vi "PEXPIREAT.vi"(8 "error in (no error)":errorcluster, 9 "expire time":timestamp, 10 "key":string, 11 "Redis Client in":refnum<class "Redis Client.lvclass">) -> (0 "error out":errorcluster, 2 "expire set?":bool, 3 "Redis Client out":refnum<class "Redis Client.lvclass">)   [LabVIEW 2019, in "Redis Client for LabVIEW.lvlib" / "Redis Client.lvclass"]
uses:
  Redis Client.lvclass
  lib/RESP3-for-LabVIEW/RESP3/subVIs/RESP3 Make String Base.vi
  lib/RESP3-for-LabVIEW/RESP3/types/RESP3 data type attribute.vi
  lib/RESP3-for-LabVIEW/RESP3/high-level/RESP3 Make Array.vi
  lib/RESP3-for-LabVIEW/RESP3/high-level/RESP3 Get String.vi
  lib/RESP3-for-LabVIEW/RESP3/high-level/RESP3 Get Integer.vi
  lib/RESP3-for-LabVIEW/RESP3/RESP3.lvlib
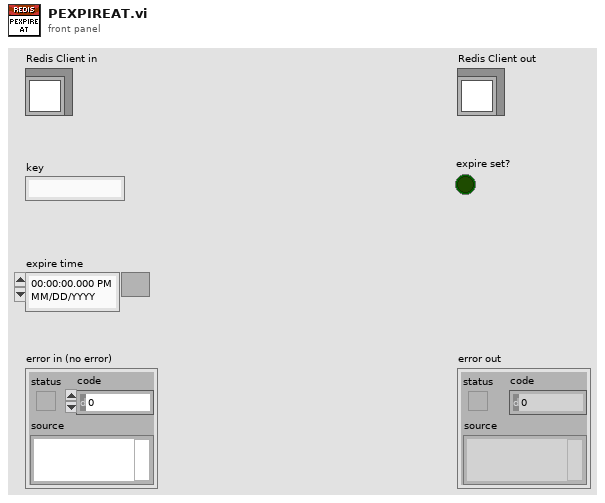
[diagram p1: front panel]
types:
  T1 = typedef "RESP3.lvlib/RESP3 Type.ctl" = enum8{"<0x00>", "<0x01>", "<0x02>", "<0x03>", "<0x04>", "<0x05>", "<0x06>", "<0x07>", "<0x08>", "<0x09>", "<0x0A>", "<0x0B>", "<0x0C>", "<0x0D>", "<0x0E>", "<0x0F>", "<0x10>", "<0x11>", "<0x12>", "<0x13>", "<0x14>", "<0x15>", "<0x16>", "<0x17>", "<0x18>", "<0x19>", "<0x1A>", "<0x1B>", "<0x1C>", "<0x1D>", "<0x1E>", "<0x1F>", "\" \"", "BLOB ERROR", "\"\"\"", "BOOLEAN", "BLOB", "MAP", "\"&\"", "\"'\"", "BIG NUMBER", "\")\"", "ARRAY", "STRING", "DOUBLE", "ERROR", "END", "\"/\"", "\"0\"", "\"1\"", "\"2\"", "\"3\"", "\"4\"", "\"5\"", "\"6\"", "\"7\"", "\"8\"", "\"9\"", "INTEGER", "STREAM", "\"<\"", "VERBATIM STRING", "PUSH", "\"?\"", "\"@\"", "\"A\"", "\"B\"", "\"C\"", "\"D\"", "\"E\"", "\"F\"", "\"G\"", "\"H\"", "\"I\"", "\"J\"", "\"K\"", "\"L\"", "\"M\"", "\"N\"", "\"O\"", "\"P\"", "\"Q\"", "\"R\"", "\"S\"", "\"T\"", "\"U\"", "\"V\"", "\"W\"", "\"X\"", "\"Y\"", "\"Z\"", "\"[\"", "\"\\\"", "\"]\"", "\"^\"", "NULL", "\"`\"", "\"a\"", "\"b\"", "\"c\"", "\"d\"", "\"e\"", "\"f\"", "\"g\"", "\"h\"", "\"i\"", "\"j\"", "\"k\"", "\"l\"", "\"m\"", "\"n\"", "\"o\"", "\"p\"", "\"q\"", "\"r\"", "\"s\"", "\"t\"", "\"u\"", "\"v\"", "\"w\"", "\"x\"", "\"y\"", "\"z\"", "\"{\"", "ATTRIBUTES", "\"}\"", "SET", "<0x7F>", "<0x80>", "<0x81>", "<0x82>", "<0x83>", "<0x84>", "<0x85>", "<0x86>", "<0x87>", "<0x88>", "<0x89>", "<0x8A>", "<0x8B>", "<0x8C>", "<0x8D>", "<0x8E>", "<0x8F>", "<0x90>", "<0x91>", "<0x92>", "<0x93>", "<0x94>", "<0x95>", "<0x96>", "<0x97>", "<0x98>", "<0x99>", "<0x9A>", "<0x9B>", "<0x9C>", "<0x9D>", "<0x9E>", "<0x9F>", "<0xA0>", "<0xA1>", "<0xA2>", "<0xA3>", "<0xA4>", "<0xA5>", "<0xA6>", "<0xA7>", "<0xA8>", "<0xA9>", "<0xAA>", "<0xAB>", "<0xAC>", "<0xAD>", "<0xAE>", "<0xAF>", "<0xB0>", "<0xB1>", "<0xB2>", "<0xB3>", "<0xB4>", "<0xB5>", "<0xB6>", "<0xB7>", "<0xB8>", "<0xB9>", "<0xBA>", "<0xBB>", "<0xBC>", "<0xBD>", "<0xBE>", "<0xBF>", "<0xC0>", "<0xC1>", "<0xC2>", "<0xC3>", "<0xC4>", "<0xC5>", "<0xC6>", "<0xC7>", "<0xC8>", "<0xC9>", "<0xCA>", "<0xCB>", "<0xCC>", "<0xCD>", "<0xCE>", "<0xCF>", "<0xD0>", "<0xD1>", "<0xD2>", "<0xD3>", "<0xD4>", "<0xD5>", "<0xD6>", "<0xD7>", "<0xD8>", "<0xD9>", "<0xDA>", "<0xDB>", "<0xDC>", "<0xDD>", "<0xDE>", "<0xDF>", "<0xE0>", "<0xE1>", "<0xE2>", "<0xE3>", "<0xE4>", "<0xE5>", "<0xE6>", "<0xE7>", "<0xE8>", "<0xE9>", "<0xEA>", "<0xEB>", "<0xEC>", "<0xED>", "<0xEE>", "<0xEF>", "<0xF0>", "<0xF1>", "<0xF2>", "<0xF3>", "<0xF4>", "<0xF5>", "<0xF6>", "<0xF7>", "<0xF8>", "<0xF9>", "<0xFA>", "<0xFB>", "<0xFC>", "<0xFD>", "<0xFE>"}
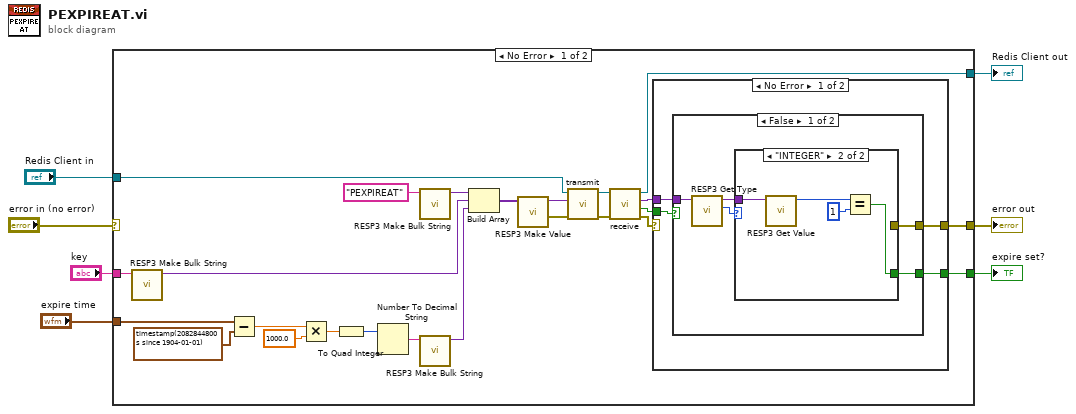
[diagram p0: block diagram]
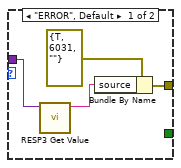
[diagram p2: hidden frame]
diagram:
  n1 = case shown="No Error" "error in (no error)" {
    selector: "error in (no error)" -> [_ w51]
    tunnel: [w29 w51] -> w6
    tunnel: "Redis Client in" -> [w31 w50]
    tunnel: [w30 w50] -> w4
    tunnel: "key" -> [w18 _]
    tunnel: [w19 _] -> w1
    tunnel: "expire time" -> [w12 _]
    frame No Error {
      n2 = call "RESP3 Make Bulk String.vi"("String"=w18) -> ("RESP3 Value out"=w17:variant)  [unwired: 9 in, 1 out]
      n3 = Subtract(x=w12, y=timestamp(2082844800 s since 1904-01-01)) -> (x-y=w11:dbl)
      n4 = Multiply(x=w11, y=1000.0) -> (x*y=w10:dbl)
      n5 = To Quad Integer(1:w10) -> (0:w8:i64)
      n6 = Number To Decimal String(number=w8) -> (decimal integer string=w15:string)  [unwired: 1 in]
      n7 = call "RESP3 Make Bulk String.vi"("String"="PEXPIREAT" ("string in")) -> ("RESP3 Value out"=w20:variant)  [unwired: 9 in, 1 out]
      n8 = call "RESP3 Make Bulk String.vi"("String"=w15) -> ("RESP3 Value out"=w16:variant)  [unwired: 9 in, 1 out]
      n9 = Build Array(w20, w17, w16) -> (w14:variant[])
      n10 = call-poly "RESP3 Make Value.vi"("RESP3 Values in"=w14) -> ("error out"=w23:errorcluster, "RESP3 Value out"=w22:variant)  [unwired: 9 in]
      n11 = call-dynamic "transmit.vi"("error in (no error)"=w23, "RESP3 Value"=w22, "Redis Client in"=w31) -> ("error out"=w27:errorcluster, "Redis Client out"=w28:refnum<class "Redis Client.lvclass">)  [unwired: 7 in]
      n12 = call-dynamic "receive.vi"("error in (no error)"=w27, "Redis Client in"=w28) -> ("error out"=w24:errorcluster, "timed out?"=w25:bool, "RESP3 Value"=w26:variant, "Redis Client out"=w30:refnum<class "Redis Client.lvclass">)  [unwired: 6 in]
      n13 = case shown="No Error" w24 {
        selector: w24 -> [_ w49]
        tunnel: [w35 w49] -> w29
        tunnel: w26 -> [w34 _]
        tunnel: w25 -> [w33 _]
        tunnel: [w32 _] -> w19
        frame No Error {
          n14 = case shown="False" w33 {
            tunnel: [w40 _] -> w35
            tunnel: w34 -> [w38 _]
            tunnel: [w36 _] -> w32
            frame False {
              n15 = call "RESP3 Get Type.vi"("RESP3 Value in"=w38) -> ("RESP3 Type"=w37:T1, "RESP3 Value out"=w39:variant)  [unwired: 7 in, 2 out]
              n16 = case shown="\"INTEGER\"" w37 {
                tunnel: [w42 _] -> w40
                tunnel: w39 -> [w41 w48]
                tunnel: [_ w45] -> w36
                frame "ERROR", Default {
                  n17 = call-poly "RESP3 Get Value.vi"("RESP3 Value in"=w41) -> ("String out"=w43:string)  [unwired: 7 in, 3 out]
                  n18 = Bundle By Name(cluster=errorcluster {"status"=TRUE, "code"=6031, "source"=""} ("error constant"), "source"=w43) -> (w42:errorcluster)
                }
                frame "INTEGER" {
                  n19 = call-poly "RESP3 Get Value.vi"("RESP3 Value in"=w48) -> ("I64 out"=w47:i64)  [unwired: 8 in, 2 out]
                  n20 = Equal?(x=w47, y=i64 1) -> (x = y?=w45:bool)
                }
              }
            }
            frame True {
            }
          }
        }
        frame Error {
        }
      }
    }
    frame Error {
    }
  }
  "error out" <- w6
  "Redis Client out" <- w4
  "expire set?" <- w1
